vi "HTML Report Filter Special Characters.vi"(10 "character string":string, 11 "HTML in":string) -> (3 "HTML out":string)   [LabVIEW 2015, in "NI_ReportGenerationCore.lvlib"]
doc: "Encodes restricted characters in \"character string\" and appends it to HTML in."
uses:
  <vilib>/Utility/NIReport.llb/NI_ReportGenerationCore.lvlib
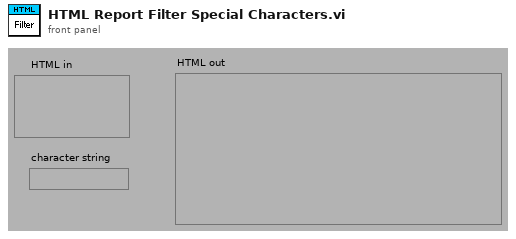
[diagram p1: front panel]
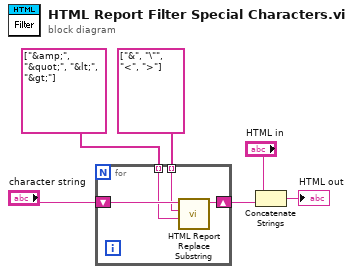
[diagram p0: block diagram]
diagram:
  n1 = for {
    shift-right: [w9] -> w1
    shift-left: "character string" -> [w10]
    tunnel: string[] ["&", "\"", "<", ">"] ("Labels") -> [w8] mode=indexing
    tunnel: string[] ["&amp;", "&quot;", "&lt;", "&gt;"] ("Labels") -> [w7] mode=indexing
    n2 = call <vilib>:"HTML Report Replace Substring.vi"("replacement"=w7, "pattern"=w8, "text"=w10) -> ("text out"=w9:string)  [unwired: 3 in, 5 out]
  }
  n3 = Concatenate Strings("HTML in", w1) -> (→"HTML out":string)
